vi "04TRM800_SendMessage.vi"(7 "Str Refnum":refnum<vi>, 8 "error in (no error)":errorcluster, 10 "String":string, 11 "Enum":enum16{"Initialize", "Send Message"}(ring)) -> (0 "error out":errorcluster)   [LabVIEW 2020]
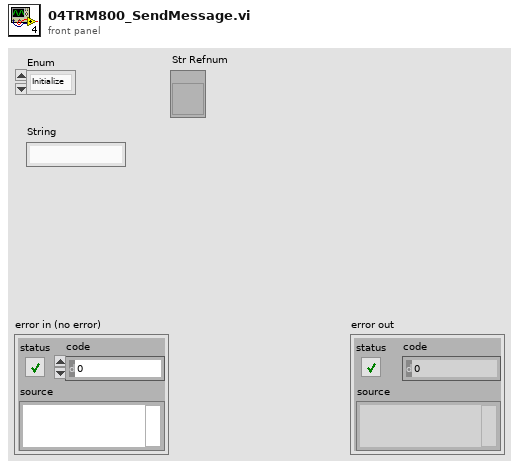
[diagram p1: front panel]
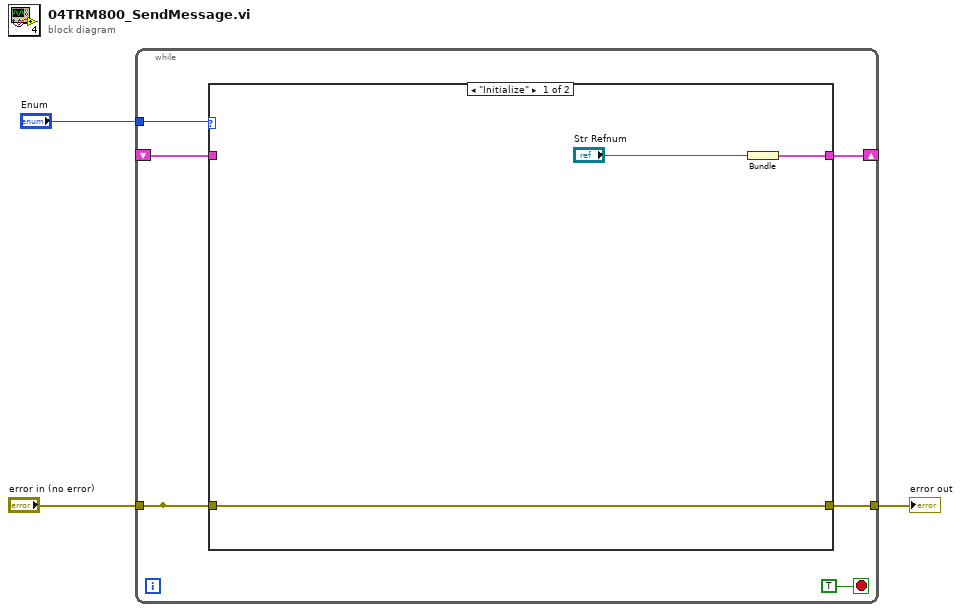
[diagram p0: block diagram]
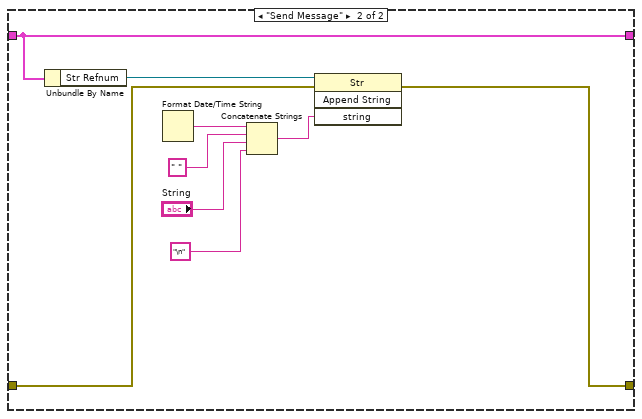
[diagram p2: hidden frame]
diagram:
  n1 = while {
    tunnel: [w9] -> _
    tunnel: "error in (no error)" -> [w9]
    tunnel: [w8] -> w2
    tunnel: "Enum" -> [w6]
    shift-right: [w5] -> _
    shift-left: _ -> [w4]
    stop <- TRUE stop-if-true
    n2 = case shown="\"Initialize\"" w6 {
      tunnel: w9 -> [w10 w19]
      tunnel: [w10 w13] -> w8
      tunnel: [w11 w21] -> w5
      tunnel: w4 -> [_ w21]
      frame "Initialize" {
        n3 = Bundle("Str Refnum"="Str Refnum") -> (w11:cluster{"Str Refnum":refnum<vi>})  [unwired: 1 in]
      }
      frame "Send Message" {
        n4 = Unbundle By Name(w21) -> ("Str Refnum"=w20:refnum<vi>)
        n5 = Format Date/Time String() -> (date/time string=w18:string)  [unwired: 3 in]
        n6 = Concatenate Strings(w18, " ", "String", "\n") -> (w14:string)
        n7 = invoke class="Str" method="Append String"(reference=w20, error in=w19, "string"=w14) -> (error out=w13:errorcluster)  [unwired: 1 in, 3 out]
      }
    }
  }
  "error out" <- w2
